vi "Read Buffer.vi"(8 "error in (no error)":errorcluster, 10 "buffer in":u8[](array[numeric]), 11 "Buffer data":T1 {"channels"."string offset" format="%d bytes"; "avg bandwidth" format="%.0g bytes"}) -> (0 "error out":errorcluster, 2 "buffer out":u8[](array[numeric]), 3 "buffer string":string, 5 "buffer size":u64, 7 "null?":bool)   [LabVIEW 2017, in "DSF Core.lvlib"]
uses:
  DSF Core.lvlib
  Buffer Data.ctl
  Classes/Buffer/Buffer.lvclass
  C:/Program Files (x86)/National Instruments/LabVIEW 2017/vi.lib/NI/Memory Manager/Classes/Pointer/Pointer.lvclass
  Classes/Transfer Group Status/Status.lvclass
  Typedefs/DSF Data Type.ctl
  Typedefs/DSF Engine Channel Configuration.ctl
  Typedefs/DSF Settings Info.ctl
  <vilib>/NI/Memory Manager/Classes/Pointer/Pointer.lvclass/Pointer.ctl
  <vilib>/NI/Memory Manager/Classes/Pointer/Get Size.vi
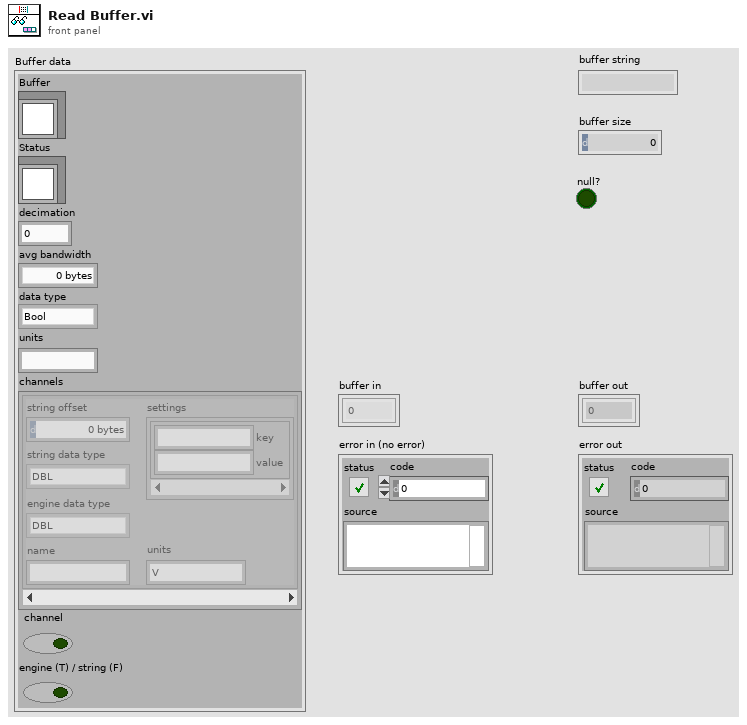
[diagram p1: front panel]
types:
  T1 = typedef "DSF Core.lvlib/Buffer Data.ctl" = cluster{"Buffer":refnum<class "Buffer.lvclass">, "Status":refnum<class "Status.lvclass">, "decimation":u64, "avg bandwidth":dbl, "data type":T2, "units":string, "channels":T3[], "channel":bool, "engine (T) / string (F)":bool}
  T2 = typedef "DSF Core.lvlib/DSF Data Type.ctl" = enum8{"Bool", "SGL", "DBL", "I8", "I16", "I32", "I64", "U8", "U16", "U32", "U64"}
  T3 = typedef "DSF Core.lvlib/DSF Engine Channel Configuration.ctl" = cluster{"string offset":u64, "string data type":T2, "engine data type":T2, "name":string, "settings":T4, "units":string}
  T4 = typedef "DSF Core.lvlib/DSF Settings Info.ctl" = cluster{"key":string, "value":string}[]
  T5 = enum16{"big-endian, network order", "native, host order", "little-endian"}
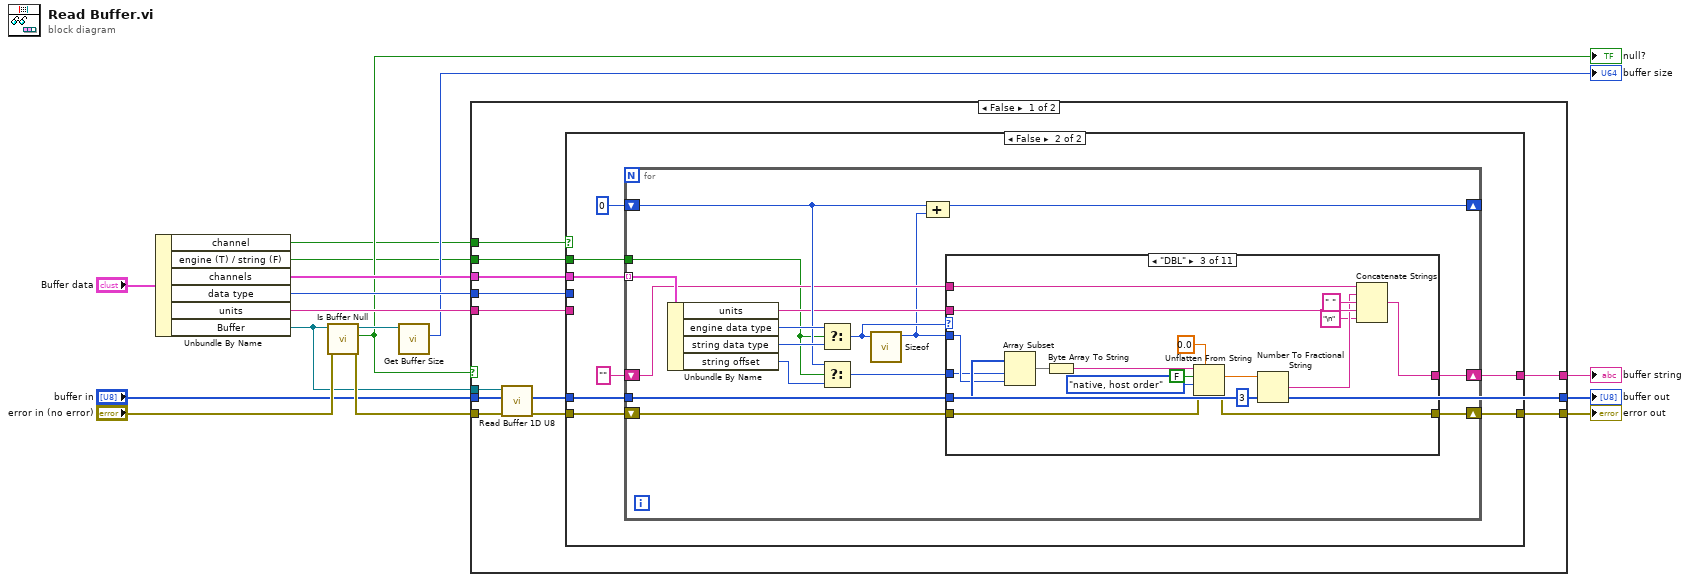
[diagram p0: block diagram]
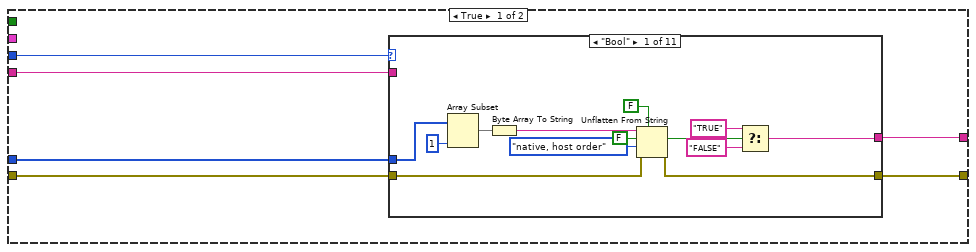
[diagram p2: hidden frame]
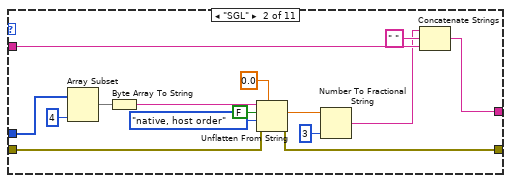
[diagram p3: hidden frame]
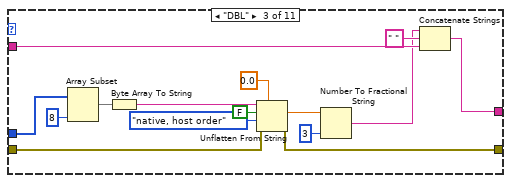
[diagram p4: hidden frame]
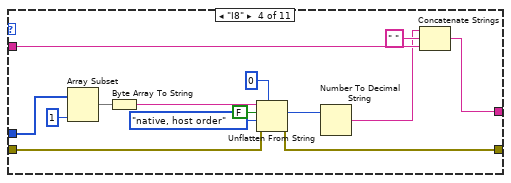
[diagram p5: hidden frame]
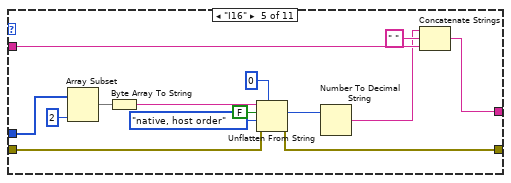
[diagram p6: hidden frame]
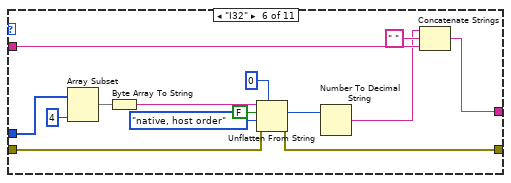
[diagram p7: hidden frame]
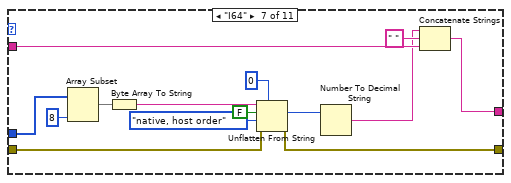
[diagram p8: hidden frame]
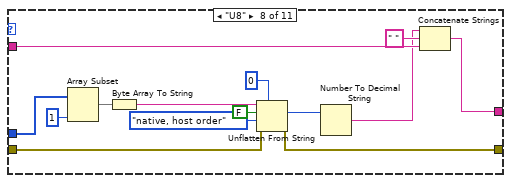
[diagram p9: hidden frame]
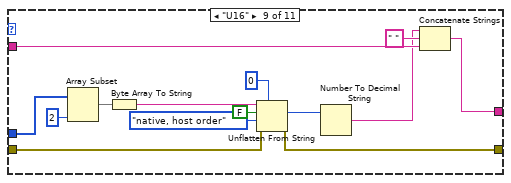
[diagram p10: hidden frame]
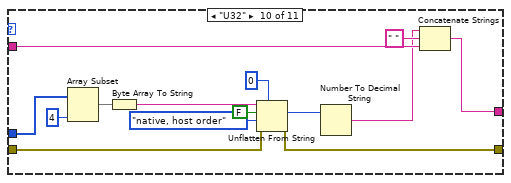
[diagram p11: hidden frame]
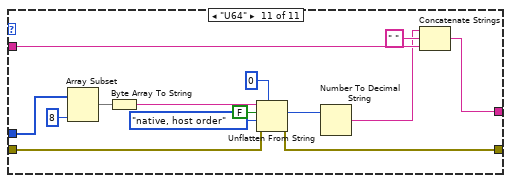
[diagram p12: hidden frame]
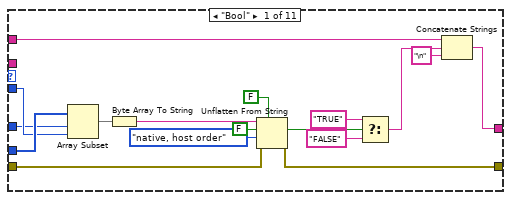
[diagram p13: hidden frame]
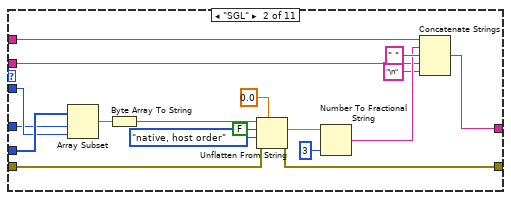
[diagram p14: hidden frame]
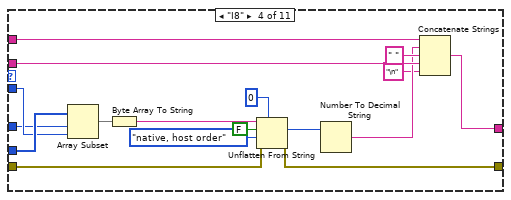
[diagram p15: hidden frame]
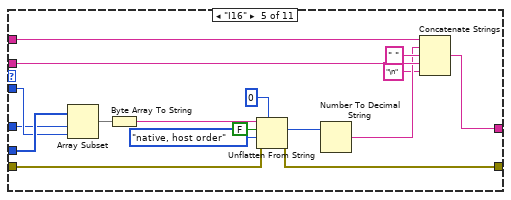
[diagram p16: hidden frame]
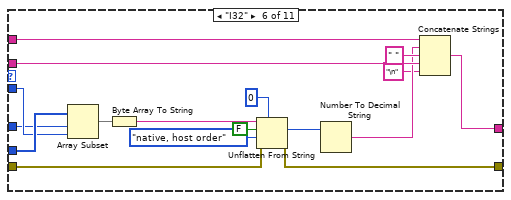
[diagram p17: hidden frame]
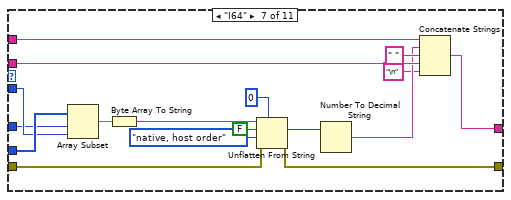
[diagram p18: hidden frame]
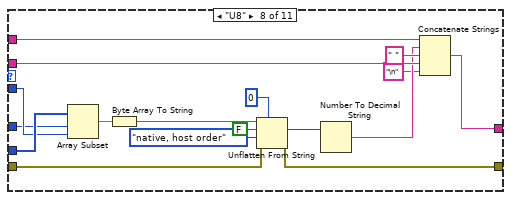
[diagram p19: hidden frame]
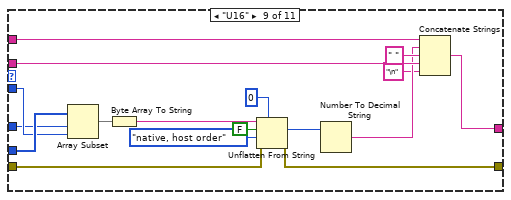
[diagram p20: hidden frame]
diagram:
  n1 = Unbundle By Name("Buffer data") -> ("channel"=w2:bool, "engine (T) / string (F)"=w1:bool, "channels"=w6:T3[], "data type"=w14:T2, "units"=w13:string, "Buffer"=w11:refnum<class "Buffer.lvclass">)
  n2 = call "Is Buffer Null.vi"("error in (no error)"="error in (no error)", "Buffer in"=w11) -> ("error out"=w12:errorcluster, "null?"=w4:bool, "Buffer out"=w16:refnum<class "Buffer.lvclass">)  [unwired: 7 in]
  "null?" <- w4
  n3 = call "Get Buffer Size.vi"("Buffer in"=w16) -> ("buffer size"=→"buffer size":u64)  [unwired: 9 in, 1 out]
  n4 = case shown="False" w4 {
    tunnel: w14 -> [w28 _]
    tunnel: w13 -> [w17 _]
    tunnel: w12 -> [w27 w403]
    tunnel: w11 -> [w26 _]
    tunnel: "buffer in" -> [w25 w405]
    tunnel: [w23 w403] -> w9
    tunnel: [w22 w405] -> w8
    tunnel: [w21 ""] -> w7
    tunnel: w2 -> [w20 _]
    tunnel: w6 -> [w19 _]
    tunnel: w1 -> [w18 _]
    frame False {
      n5 = call "Read Buffer 1D U8.vi"("error in (no error)"=w27, "dst array in"=w25, "Buffer in"=w26) -> ("error out"=w24:errorcluster, "dst array out"=w22:u8[])  [unwired: 5 in, 2 out]
      n6 = case shown="False" w20 {
        tunnel: w28 -> [w34 _]
        tunnel: w17 -> [w33 _]
        tunnel: w24 -> [w32 w197]
        tunnel: [w31 w196] -> w23
        tunnel: w22 -> [w30 w195]
        tunnel: [w29 w192] -> w21
        tunnel: w19 -> [_ w194]
        tunnel: w18 -> [_ w193]
        frame True {
          n7 = case shown="\"Bool\"" w34 {
            tunnel: w30 -> [w47 w62 w77 w91 w105 w119 w133 w147 w161 w175 w189]
            tunnel: w33 -> [_ w50 w65 w80 w94 w108 w122 w136 w150 w164 w178]
            tunnel: w32 -> [w43 w58 w73 w87 w101 w115 w129 w143 w157 w171 w185]
            tunnel: [w42 w57 w72 w86 w100 w114 w128 w142 w156 w170 w184] -> w31
            tunnel: [w35 w49 w64 w79 w93 w107 w121 w135 w149 w163 w177] -> w29
            frame "Bool" {
              n8 = Array Subset(array=w47, length=1) -> (w45:u8[])  [unwired: 1 in]
              n9 = Byte Array To String(unsigned byte array=w45) -> (string=w41:string)
              n10 = Unflatten From String(type=FALSE, binary string=w41, data includes array or string size? (T)=FALSE, byte order (0:big-endian, network order)=T5."native, host order", error in (no error)=w43) -> (value=w38:bool, error out=w42:errorcluster)  [unwired: 1 out]
              n11 = Select(t="TRUE", s=w38, f="FALSE") -> (s? t:f=w35:string)
            }
            frame "SGL" {
              n12 = Array Subset(array=w62, length=4) -> (w60:u8[])  [unwired: 1 in]
              n13 = Byte Array To String(unsigned byte array=w60) -> (string=w56:string)
              n14 = Unflatten From String(type=sgl 0.0, binary string=w56, data includes array or string size? (T)=FALSE, byte order (0:big-endian, network order)=T5."native, host order", error in (no error)=w58) -> (value=w53:sgl, error out=w57:errorcluster)  [unwired: 1 out]
              n15 = Number To Fractional String(number=w53, precision (6)=i16 3) -> (F-format string=w48:string)  [unwired: 2 in]
              n16 = Concatenate Strings(w48, " " ("string"), w50) -> (w49:string)
            }
            frame "DBL" {
              n17 = Array Subset(array=w77, length=8) -> (w75:u8[])  [unwired: 1 in]
              n18 = Byte Array To String(unsigned byte array=w75) -> (string=w71:string)
              n19 = Unflatten From String(type=0.0, binary string=w71, data includes array or string size? (T)=FALSE, byte order (0:big-endian, network order)=T5."native, host order", error in (no error)=w73) -> (value=w68:dbl, error out=w72:errorcluster)  [unwired: 1 out]
              n20 = Number To Fractional String(number=w68, precision (6)=i16 3) -> (F-format string=w63:string)  [unwired: 2 in]
              n21 = Concatenate Strings(w63, " " ("string"), w65) -> (w64:string)
            }
            frame "I8" {
              n22 = Array Subset(array=w91, length=1) -> (w89:u8[])  [unwired: 1 in]
              n23 = Byte Array To String(unsigned byte array=w89) -> (string=w85:string)
              n24 = Unflatten From String(type=i8 0, binary string=w85, data includes array or string size? (T)=FALSE, byte order (0:big-endian, network order)=T5."native, host order", error in (no error)=w87) -> (value=w82:i8, error out=w86:errorcluster)  [unwired: 1 out]
              n25 = Number To Decimal String(number=w82) -> (decimal integer string=w78:string)  [unwired: 1 in]
              n26 = Concatenate Strings(w78, " " ("string"), w80) -> (w79:string)
            }
            frame "I16" {
              n27 = Array Subset(array=w105, length=2) -> (w103:u8[])  [unwired: 1 in]
              n28 = Byte Array To String(unsigned byte array=w103) -> (string=w99:string)
              n29 = Unflatten From String(type=i16 0, binary string=w99, data includes array or string size? (T)=FALSE, byte order (0:big-endian, network order)=T5."native, host order", error in (no error)=w101) -> (value=w96:i16, error out=w100:errorcluster)  [unwired: 1 out]
              n30 = Number To Decimal String(number=w96) -> (decimal integer string=w92:string)  [unwired: 1 in]
              n31 = Concatenate Strings(w92, " " ("string"), w94) -> (w93:string)
            }
            frame "I32" {
              n32 = Array Subset(array=w119, length=4) -> (w117:u8[])  [unwired: 1 in]
              n33 = Byte Array To String(unsigned byte array=w117) -> (string=w113:string)
              n34 = Unflatten From String(type=0, binary string=w113, data includes array or string size? (T)=FALSE, byte order (0:big-endian, network order)=T5."native, host order", error in (no error)=w115) -> (value=w110:i32, error out=w114:errorcluster)  [unwired: 1 out]
              n35 = Number To Decimal String(number=w110) -> (decimal integer string=w106:string)  [unwired: 1 in]
              n36 = Concatenate Strings(w106, " " ("string"), w108) -> (w107:string)
            }
            frame "I64" {
              n37 = Array Subset(array=w133, length=8) -> (w131:u8[])  [unwired: 1 in]
              n38 = Byte Array To String(unsigned byte array=w131) -> (string=w127:string)
              n39 = Unflatten From String(type=i64 0, binary string=w127, data includes array or string size? (T)=FALSE, byte order (0:big-endian, network order)=T5."native, host order", error in (no error)=w129) -> (value=w124:i64, error out=w128:errorcluster)  [unwired: 1 out]
              n40 = Number To Decimal String(number=w124) -> (decimal integer string=w120:string)  [unwired: 1 in]
              n41 = Concatenate Strings(w120, " " ("string"), w122) -> (w121:string)
            }
            frame "U8" {
              n42 = Array Subset(array=w147, length=1) -> (w145:u8[])  [unwired: 1 in]
              n43 = Byte Array To String(unsigned byte array=w145) -> (string=w141:string)
              n44 = Unflatten From String(type=u8 0, binary string=w141, data includes array or string size? (T)=FALSE, byte order (0:big-endian, network order)=T5."native, host order", error in (no error)=w143) -> (value=w138:u8, error out=w142:errorcluster)  [unwired: 1 out]
              n45 = Number To Decimal String(number=w138) -> (decimal integer string=w134:string)  [unwired: 1 in]
              n46 = Concatenate Strings(w134, " " ("string"), w136) -> (w135:string)
            }
            frame "U16" {
              n47 = Array Subset(array=w161, length=2) -> (w159:u8[])  [unwired: 1 in]
              n48 = Byte Array To String(unsigned byte array=w159) -> (string=w155:string)
              n49 = Unflatten From String(type=u16 0, binary string=w155, data includes array or string size? (T)=FALSE, byte order (0:big-endian, network order)=T5."native, host order", error in (no error)=w157) -> (value=w152:u16, error out=w156:errorcluster)  [unwired: 1 out]
              n50 = Number To Decimal String(number=w152) -> (decimal integer string=w148:string)  [unwired: 1 in]
              n51 = Concatenate Strings(w148, " " ("string"), w150) -> (w149:string)
            }
            frame "U32" {
              n52 = Array Subset(array=w175, length=4) -> (w173:u8[])  [unwired: 1 in]
              n53 = Byte Array To String(unsigned byte array=w173) -> (string=w169:string)
              n54 = Unflatten From String(type=u32 0, binary string=w169, data includes array or string size? (T)=FALSE, byte order (0:big-endian, network order)=T5."native, host order", error in (no error)=w171) -> (value=w166:u32, error out=w170:errorcluster)  [unwired: 1 out]
              n55 = Number To Decimal String(number=w166) -> (decimal integer string=w162:string)  [unwired: 1 in]
              n56 = Concatenate Strings(w162, " " ("string"), w164) -> (w163:string)
            }
            frame "U64" {
              n57 = Array Subset(array=w189, length=8) -> (w187:u8[])  [unwired: 1 in]
              n58 = Byte Array To String(unsigned byte array=w187) -> (string=w183:string)
              n59 = Unflatten From String(type=u64 0, binary string=w183, data includes array or string size? (T)=FALSE, byte order (0:big-endian, network order)=T5."native, host order", error in (no error)=w185) -> (value=w180:u64, error out=w184:errorcluster)  [unwired: 1 out]
              n60 = Number To Decimal String(number=w180) -> (decimal integer string=w176:string)  [unwired: 1 in]
              n61 = Concatenate Strings(w176, " " ("string"), w178) -> (w177:string)
            }
          }
        }
        frame False {
          n62 = for {
            tunnel: w195 -> [w211]
            shift-right: [w212] -> w196
            shift-left: w197 -> [w213]
            tunnel: w194 -> [w210] mode=indexing
            tunnel: w193 -> [w198]
            shift-right: [w203] -> w192
            shift-left: "" -> [w201]
            shift-right: [w204] -> _
            shift-left: u64 0 -> [w205]
            n63 = Unbundle By Name(w210) -> ("units"=w202:string, "engine data type"=w206:T2, "string data type"=w207:T2, "string offset"=w209:u64)
            n64 = Select(t=w206, s=w198, f=w207) -> (s? t:f=w200:T2)
            n65 = Select(t=w205, s=w198, f=w209) -> (s? t:f=w208:u64)
            n66 = call "Sizeof.vi"("data type"=w200) -> ("size in bytes"=w199:u64)  [unwired: 9 in, 1 out]
            n67 = Compound Arithmetic op=ADD(w205, w199) -> (w204:u64)
            n68 = case shown="\"DBL\"" w200 {
              tunnel: w211 -> [w230 w248 w266 w283 w300 w317 w334 w351 w368 w385 w402]
              tunnel: w202 -> [_ w233 w255 w273 w290 w307 w324 w341 w358 w375 w392]
              tunnel: w213 -> [w227 w245 w263 w280 w297 w314 w331 w348 w365 w382 w399]
              tunnel: [w226 w244 w262 w279 w296 w313 w330 w347 w364 w381 w398] -> w212
              tunnel: [w217 w237 w254 w272 w289 w306 w323 w340 w357 w374 w391] -> w203
              tunnel: w208 -> [w214 w231 w249 w267 w284 w301 w318 w335 w352 w369 w389]
              tunnel: w199 -> [w215 w232 w250 w268 w285 w302 w319 w336 w353 w370 w386]
              tunnel: w201 -> [w219 w235 w252 w270 w287 w304 w321 w338 w355 w372 w388]
              frame "Bool" {
                n69 = Array Subset(array=w230, index=w214, length=w215) -> (w229:u8[])
                n70 = Byte Array To String(unsigned byte array=w229) -> (string=w225:string)
                n71 = Unflatten From String(type=FALSE, binary string=w225, data includes array or string size? (T)=FALSE, byte order (0:big-endian, network order)=T5."native, host order", error in (no error)=w227) -> (value=w222:bool, error out=w226:errorcluster)  [unwired: 1 out]
                n72 = Select(t="TRUE", s=w222, f="FALSE") -> (s? t:f=w218:string)
                n73 = Concatenate Strings(w219, w218, "\n" ("string")) -> (w217:string)
              }
              frame "SGL" {
                n74 = Array Subset(array=w248, index=w231, length=w232) -> (w247:u8[])
                n75 = Byte Array To String(unsigned byte array=w247) -> (string=w243:string)
                n76 = Unflatten From String(type=sgl 0.0, binary string=w243, data includes array or string size? (T)=FALSE, byte order (0:big-endian, network order)=T5."native, host order", error in (no error)=w245) -> (value=w240:sgl, error out=w244:errorcluster)  [unwired: 1 out]
                n77 = Number To Fractional String(number=w240, precision (6)=i16 3) -> (F-format string=w236:string)  [unwired: 2 in]
                n78 = Concatenate Strings(w235, w236, " " ("string"), w233, "\n" ("string")) -> (w237:string)
              }
              frame "DBL" {
                n79 = Array Subset(array=w266, index=w249, length=w250) -> (w265:u8[])
                n80 = Byte Array To String(unsigned byte array=w265) -> (string=w261:string)
                n81 = Unflatten From String(type=0.0, binary string=w261, data includes array or string size? (T)=FALSE, byte order (0:big-endian, network order)=T5."native, host order", error in (no error)=w263) -> (value=w258:dbl, error out=w262:errorcluster)  [unwired: 1 out]
                n82 = Number To Fractional String(number=w258, precision (6)=i16 3) -> (F-format string=w253:string)  [unwired: 2 in]
                n83 = Concatenate Strings(w252, w253, " " ("string"), w255, "\n" ("string")) -> (w254:string)
              }
              frame "I8" {
                n84 = Array Subset(array=w283, index=w267, length=w268) -> (w282:u8[])
                n85 = Byte Array To String(unsigned byte array=w282) -> (string=w278:string)
                n86 = Unflatten From String(type=i8 0, binary string=w278, data includes array or string size? (T)=FALSE, byte order (0:big-endian, network order)=T5."native, host order", error in (no error)=w280) -> (value=w275:i8, error out=w279:errorcluster)  [unwired: 1 out]
                n87 = Number To Decimal String(number=w275) -> (decimal integer string=w271:string)  [unwired: 1 in]
                n88 = Concatenate Strings(w270, w271, " " ("string"), w273, "\n" ("string")) -> (w272:string)
              }
              frame "I16" {
                n89 = Array Subset(array=w300, index=w284, length=w285) -> (w299:u8[])
                n90 = Byte Array To String(unsigned byte array=w299) -> (string=w295:string)
                n91 = Unflatten From String(type=i16 0, binary string=w295, data includes array or string size? (T)=FALSE, byte order (0:big-endian, network order)=T5."native, host order", error in (no error)=w297) -> (value=w292:i16, error out=w296:errorcluster)  [unwired: 1 out]
                n92 = Number To Decimal String(number=w292) -> (decimal integer string=w288:string)  [unwired: 1 in]
                n93 = Concatenate Strings(w287, w288, " " ("string"), w290, "\n" ("string")) -> (w289:string)
              }
              frame "I32" {
                n94 = Array Subset(array=w317, index=w301, length=w302) -> (w316:u8[])
                n95 = Byte Array To String(unsigned byte array=w316) -> (string=w312:string)
                n96 = Unflatten From String(type=0, binary string=w312, data includes array or string size? (T)=FALSE, byte order (0:big-endian, network order)=T5."native, host order", error in (no error)=w314) -> (value=w309:i32, error out=w313:errorcluster)  [unwired: 1 out]
                n97 = Number To Decimal String(number=w309) -> (decimal integer string=w305:string)  [unwired: 1 in]
                n98 = Concatenate Strings(w304, w305, " " ("string"), w307, "\n" ("string")) -> (w306:string)
              }
              frame "I64" {
                n99 = Array Subset(array=w334, index=w318, length=w319) -> (w333:u8[])
                n100 = Byte Array To String(unsigned byte array=w333) -> (string=w329:string)
                n101 = Unflatten From String(type=i64 0, binary string=w329, data includes array or string size? (T)=FALSE, byte order (0:big-endian, network order)=T5."native, host order", error in (no error)=w331) -> (value=w326:i64, error out=w330:errorcluster)  [unwired: 1 out]
                n102 = Number To Decimal String(number=w326) -> (decimal integer string=w322:string)  [unwired: 1 in]
                n103 = Concatenate Strings(w321, w322, " " ("string"), w324, "\n" ("string")) -> (w323:string)
              }
              frame "U8" {
                n104 = Array Subset(array=w351, index=w335, length=w336) -> (w350:u8[])
                n105 = Byte Array To String(unsigned byte array=w350) -> (string=w346:string)
                n106 = Unflatten From String(type=u8 0, binary string=w346, data includes array or string size? (T)=FALSE, byte order (0:big-endian, network order)=T5."native, host order", error in (no error)=w348) -> (value=w343:u8, error out=w347:errorcluster)  [unwired: 1 out]
                n107 = Number To Decimal String(number=w343) -> (decimal integer string=w339:string)  [unwired: 1 in]
                n108 = Concatenate Strings(w338, w339, " " ("string"), w341, "\n" ("string")) -> (w340:string)
              }
              frame "U16" {
                n109 = Array Subset(array=w368, index=w352, length=w353) -> (w367:u8[])
                n110 = Byte Array To String(unsigned byte array=w367) -> (string=w363:string)
                n111 = Unflatten From String(type=u16 0, binary string=w363, data includes array or string size? (T)=FALSE, byte order (0:big-endian, network order)=T5."native, host order", error in (no error)=w365) -> (value=w360:u16, error out=w364:errorcluster)  [unwired: 1 out]
                n112 = Number To Decimal String(number=w360) -> (decimal integer string=w356:string)  [unwired: 1 in]
                n113 = Concatenate Strings(w355, w356, " " ("string"), w358, "\n" ("string")) -> (w357:string)
              }
              frame "U32" {
                n114 = Array Subset(array=w385, index=w369, length=w370) -> (w384:u8[])
                n115 = Byte Array To String(unsigned byte array=w384) -> (string=w380:string)
                n116 = Unflatten From String(type=u32 0, binary string=w380, data includes array or string size? (T)=FALSE, byte order (0:big-endian, network order)=T5."native, host order", error in (no error)=w382) -> (value=w377:u32, error out=w381:errorcluster)  [unwired: 1 out]
                n117 = Number To Decimal String(number=w377) -> (decimal integer string=w373:string)  [unwired: 1 in]
                n118 = Concatenate Strings(w372, w373, " " ("string"), w375, "\n" ("string")) -> (w374:string)
              }
              frame "U64" {
                n119 = Array Subset(array=w402, index=w389, length=w386) -> (w401:u8[])
                n120 = Byte Array To String(unsigned byte array=w401) -> (string=w397:string)
                n121 = Unflatten From String(type=u64 0, binary string=w397, data includes array or string size? (T)=FALSE, byte order (0:big-endian, network order)=T5."native, host order", error in (no error)=w399) -> (value=w394:u64, error out=w398:errorcluster)  [unwired: 1 out]
                n122 = Number To Decimal String(number=w394) -> (decimal integer string=w390:string)  [unwired: 1 in]
                n123 = Concatenate Strings(w388, w390, " " ("string"), w392, "\n" ("string")) -> (w391:string)
              }
            }
          }
        }
      }
    }
    frame True {
    }
  }
  "error out" <- w9
  "buffer out" <- w8
  "buffer string" <- w7
